vi "Emballage_BDD_heure en dixieme de sec.vi"() -> (2 "chaîne de date/heure avec dixieme de sec":string, 3 "chaîne de date/heure":string)   [LabVIEW 2020]
panel:
  out "dixieme de seconde":dbl
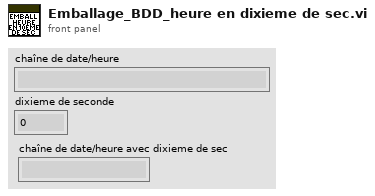
[diagram p1: front panel]
types:
  T1 = typedef "LVDateTimeRec.ctl" = cluster{"fraction de seconde":dbl, "seconde":i32, "minute":i32, "heure":i32, "jour du mois":i32, "mois":i32, "année":i32, "jour de la semaine":i32, "jour de l'année":i32, "DST":i32}
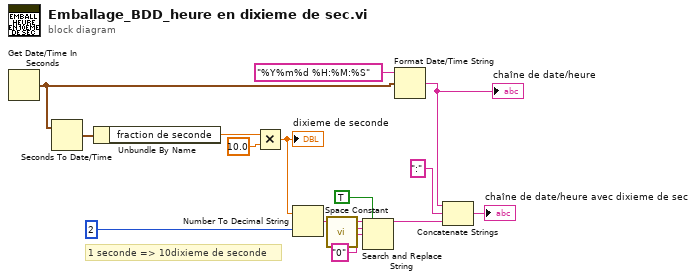
[diagram p0: block diagram]
diagram:
  # "1 seconde => 10dixieme de seconde"
  n1 = Get Date/Time In Seconds() -> (seconds since 1Jan1904=w14:timestamp)
  n2 = Seconds To Date/Time(time stamp (now)=w14) -> (date time rec=w13:T1)  [unwired: 1 in]
  n3 = Unbundle By Name(w13) -> ("fraction de seconde"=w12:dbl)
  n4 = Multiply(x=w12, y=10.0) -> (x*y=w8:dbl)
  "dixieme de seconde" <- w8
  n5 = Number To Decimal String(number=w8, width (-)=i16 2 ("largeur (-)")) -> (decimal integer string=w4:string)
  n6 = call <vilib>:"Space Constant.vi"() -> ("String"=w3:string)
  n7 = Search and Replace String(replace all?=TRUE ("tout remplacer ? (F)"), input string=w4, search string=w3, replace string="0" ("chaîne de remplacement (\"\")")) -> (result string=w5:string)  [unwired: 4 in, 3 out]
  n8 = Format Date/Time String(time format string (%c)="%Y%m%d %H:%M:%S" ("chaîne de format de l'heure (%c)"), seconds (now)=w14) -> (date/time string=w10:string)  [unwired: 1 in]
  "chaîne de date/heure" <- w10
  n9 = Concatenate Strings(w10, ":" ("chaîne"), w5) -> (→"chaîne de date/heure avec dixieme de sec":string)
